vi "Is Muted.vi"(7 "Direction":T1, 8 "error in (no error)":errorcluster, 10 "Index":i32, 11 "VMR in":refnum<class "VMR.lvclass">) -> (0 "error out":errorcluster, 2 "Muted":bool, 3 "VMR out":refnum<class "VMR.lvclass">)   [LabVIEW 2022 SP3, in "VMR-Deck.lvlib" / "VMR.lvclass"]
uses:
  VMR.lvclass
  <vilib>/IlluminatedG/IG VoicemeeterRemote API/VoiceMeeterRemote/Direction.ctl
  VMR.lvclass/VMR.ctl
  <vilib>/IlluminatedG/IG VoicemeeterRemote API/VoiceMeeterRemote/VoiceMeeterRemote/VoiceMeeterRemote.lvclass
  <vilib>/IlluminatedG/IG VoicemeeterRemote API/VoiceMeeterRemote/VoiceMeeterRemote.lvlib
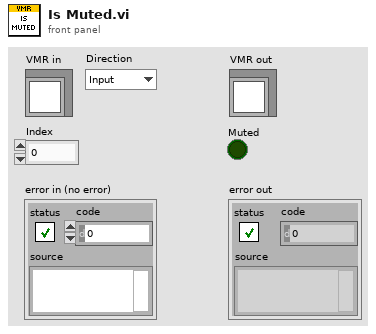
[diagram p1: front panel]
types:
  T1 = typedef "VoiceMeeterRemote.lvlib/Direction.ctl" = enum16{"Input", "Output"}
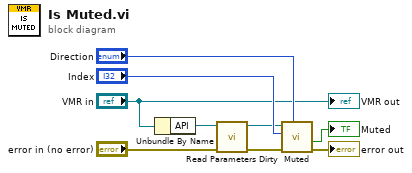
[diagram p0: block diagram]
diagram:
  n1 = Unbundle By Name("VMR in") -> ("API"=w2:refnum<class "VoiceMeeterRemote.lvclass">)
  n2 = call <vilib>:"Read Parameters Dirty.vi"("error in (no error)"="error in (no error)", "VoiceMeeterRemote in"=w2) -> ("error out"=w3:errorcluster, "VoiceMeeterRemote out"=w1:refnum<class "VoiceMeeterRemote.lvclass">)  [unwired: 7 in, 1 out]
  n3 = call <vilib>:"Muted.vi"("Direction"="Direction", "error in (no error)"=w3, "Index"="Index", "VoiceMeeterRemote in"=w1) -> ("error out"=→"error out":errorcluster, "Muted?"=→"Muted":bool)  [unwired: 5 in, 1 out]
  "VMR out" <- "VMR in"
